vi "Offsite variable.vi"() -> ()   [LabVIEW 2010]
panel:
  in  "Onsite?":u16
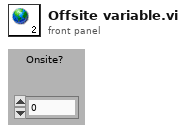
[diagram p1: front panel]
diagram:
